vi "50.vi"() -> ()   [LabVIEW 2018]
panel:
  in  "Color":string[](array[string])
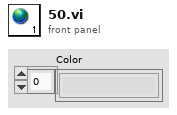
[diagram p1: front panel]
diagram:
